vi "MakeOneCycleMacro.vi"(11 "TestCycleParameters":T1={"TAmb"=20.0, "HeaterTestTemp"=-80.0, "HeaterTestDwell(min)"=30, "HeaterTestDuration"=15, "MinOpTemp"=50.0, "MinOpDwell(min)"=30, "TestHeatingRate (deg/min)"=0.4, "SurviveCycleParameters"={"MinSurviveTemp"=-131.5, "MinSurvive Dwell(min)"=10, "MaxSurviveTemp"=50.0, "MaxSurviveDwell(min)"=30, "ControlInput"=2, "ColdStandOff"=4.0, "HotStandoff"=5.0, "SteadyPWM"=20, "MaxCoolingRate (deg/min)"=4.0, "MaxHeatingRate (deg/min)"=2.5}, "CycleType"=0, "MaxOpTemp"=50.0, "MaxOpDwell(min)"=30} {"CycleType" items=["Survival", "Operational"]; "SurviveCycleParameters"."SteadyPWM" min=0 max=100 step=1; "SurviveCycleParameters"."ControlInput" items=["3A", "3B", "3C", "3D", "4A", "4B", "4C", "4D"]}) -> (2 "Profile Graph":cluster{dbl[], dbl[]}, 3 "Macro Code":string)   [LabVIEW 2024]
uses:
  controls/TestCycleParams.ctl
  controls/SurviveCycleParams.ctl
  controls/ControlInput.ctl
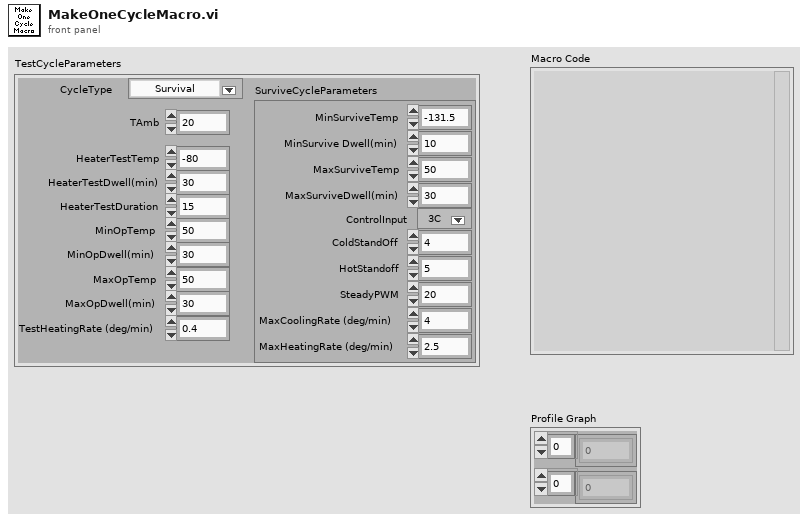
[diagram p1: front panel]
types:
  T1 = typedef "TestCycleParams.ctl" = cluster{"TAmb":dbl, "HeaterTestTemp":dbl, "HeaterTestDwell(min)":i32, "HeaterTestDuration":i32, "MinOpTemp":dbl, "MinOpDwell(min)":i32, "TestHeatingRate (deg/min)":dbl, "SurviveCycleParameters":T2, "CycleType":u16, "MaxOpTemp":dbl, "MaxOpDwell(min)":i32}
  T2 = typedef "SurviveCycleParams.ctl" = cluster{"MinSurviveTemp":dbl, "MinSurvive Dwell(min)":i32, "MaxSurviveTemp":dbl, "MaxSurviveDwell(min)":i32, "ControlInput":T3, "ColdStandOff":dbl, "HotStandoff":dbl, "SteadyPWM":i32, "MaxCoolingRate (deg/min)":dbl, "MaxHeatingRate (deg/min)":dbl}
  T3 = typedef "ControlInput.ctl" = u16
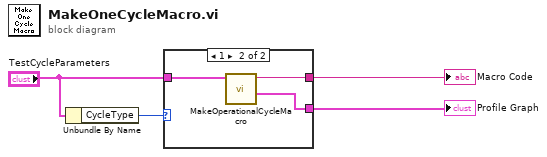
[diagram p0: block diagram]
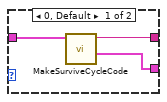
[diagram p2: hidden frame]
diagram:
  n1 = Unbundle By Name("TestCycleParameters") -> ("CycleType"=w2:u16)
  n2 = case shown="1" w2 {
    tunnel: [w7 w10] -> w3
    tunnel: "TestCycleParameters" -> [w6 w9]
    tunnel: [w5 w8] -> w4
    frame 0, Default {
      n3 = call "MakeSurviveCycleCode.vi"("TestCycleParameters"=w6) -> ("Profile"=w5:cluster{dbl[], dbl[]}, "resulting string"=w7:string)  [unwired: 9 in]
    }
    frame 1 {
      n4 = call "MakeOperationalCycleMacro.vi"("TestCycleParameters"=w9) -> ("Profile"=w8:cluster{dbl[], dbl[]}, "resulting string"=w10:string)  [unwired: 9 in]
    }
  }
  "Profile Graph" <- w4
  "Macro Code" <- w3
